vi "Get Measurement Details.vi"(8 "error in":errorcluster) -> (0 "error out":errorcluster, 1 "Measurement Annotations":T1[](array[typedef]), 2 "Service Class":string, 3 "Measurement Details":T2)   [LabVIEW 2020, in "NI-SCOPE Acquire Waveform.lvlib"]
uses:
  NI-SCOPE Acquire Waveform.lvlib
  <vilib>/MeasurementLink/MeasurementLink Measurement Server/Helpers/TypeDefs/MeasurementDetails.ctl
  <vilib>/MeasurementLink/MeasurementLink Measurement Server/Helpers/TypeDefs/MeasurementAnnotation.ctl
  <vilib>/MeasurementLink/MeasurementLink Measurement Server/MeasurementLink Measurement Server.lvlib
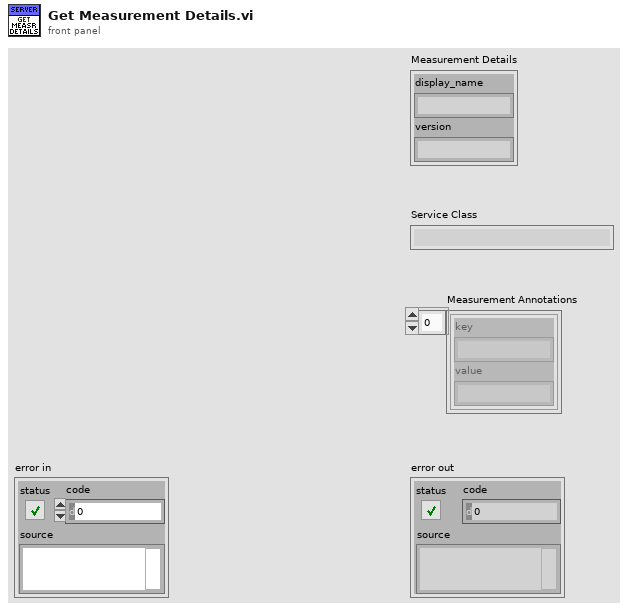
[diagram p1: front panel]
types:
  T1 = typedef "MeasurementLink Measurement Server.lvlib/MeasurementAnnotation.ctl" = cluster{"key":string, "value":string}
  T2 = typedef "MeasurementLink Measurement Server.lvlib/MeasurementDetails.ctl" = cluster{"display_name":string, "version":string}
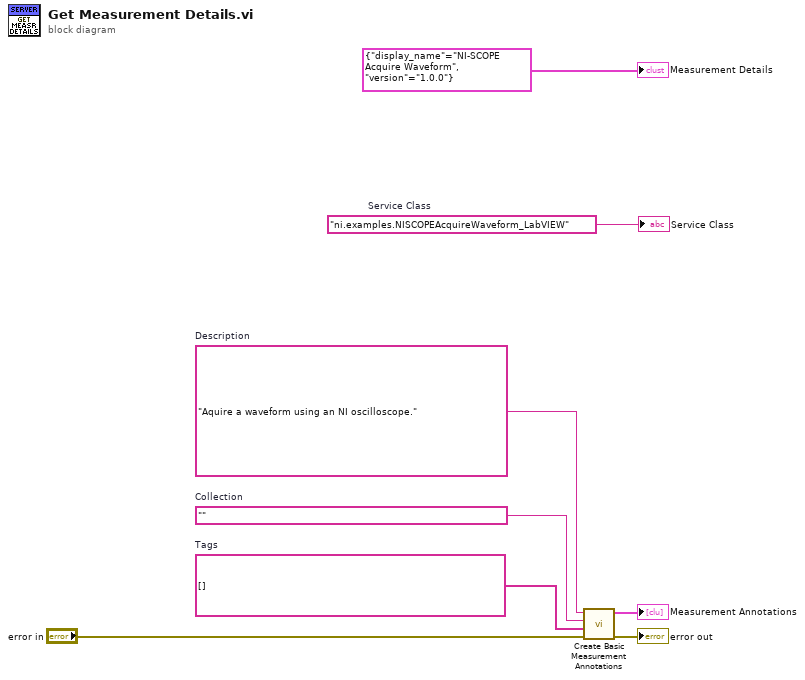
[diagram p0: block diagram]
diagram:
  w1 = string[] []  # Tags
  w2 = ""  # Collection
  w3 = "Aquire a waveform using an NI oscilloscope."  # Description
  w8 = "ni.examples.NISCOPEAcquireWaveform_LabVIEW"  # Service Class
  n1 = call <vilib>:"Create Basic Measurement Annotations.vi"("error in"="error in", "Tags"=w1, "Collection"=w2, "Description"=w3) -> ("error out"=→"error out":errorcluster, "Measurement Annotations"=→"Measurement Annotations":T1[])  [unwired: 6 in]
  "Measurement Details" <- T2 {"display_name"="NI-SCOPE Acquire Waveform", "version"="1.0.0"} ("Measurement Details")
  "Service Class" <- w8
